vi "Second Window.vi"(1 "Input Camera Image":T1(plugin-control)) -> ()   [LabVIEW 2015]
panel:
  out "Camera Image":T1(plugin-control)
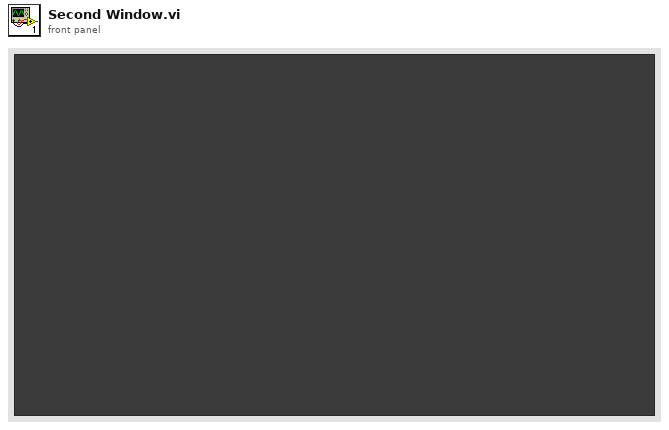
[diagram p1: front panel]
types:
  T1 = typedef "IMAQ Image.ctl" = refnum<image>
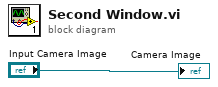
[diagram p0: block diagram]
diagram:
  "Camera Image" <- "Input Camera Image"
